vi "Read_raw_inst_setup.vi"(0 "Setup file":string) -> (8 "Setup string":string, 10 "Ch & spans choices":T2[](array[typedef]) {"Fs" format="%#_pHz"; "syncDelay" format="%#_gms"; "Ch" min=0 step=1}, 13 "PWA Data":T1, 14 "Number of Analogue instruments":i32=1, 15 "Setup filename out":string, 16 "LDA data":enum16{"No LDA data", "Take LDA data"}(ring)=enum."Take LDA data", 19 "Use Analogue channel to software sync with LDA":bool)   [LabVIEW 2022 SP3]
uses:
  Controls/Meas input Cluster.ctl
  Controls/Inst_type.ctl
  Controls/portOrDev.ctl
  Controls/calType.ctl
  Controls/channelState.ctl
  Controls/PWA_Data.ctl
  Controls/Post_Process.ctl
  File/Setup_Filetype.ctl
  Controls/Trigger_Mode.ctl
  Controls/Initial Positions.ctl
  Controls/Tunnel_Coordinates.ctl
  Globals/Meas_global.vi
  Globals/Trav_pos_global.vi
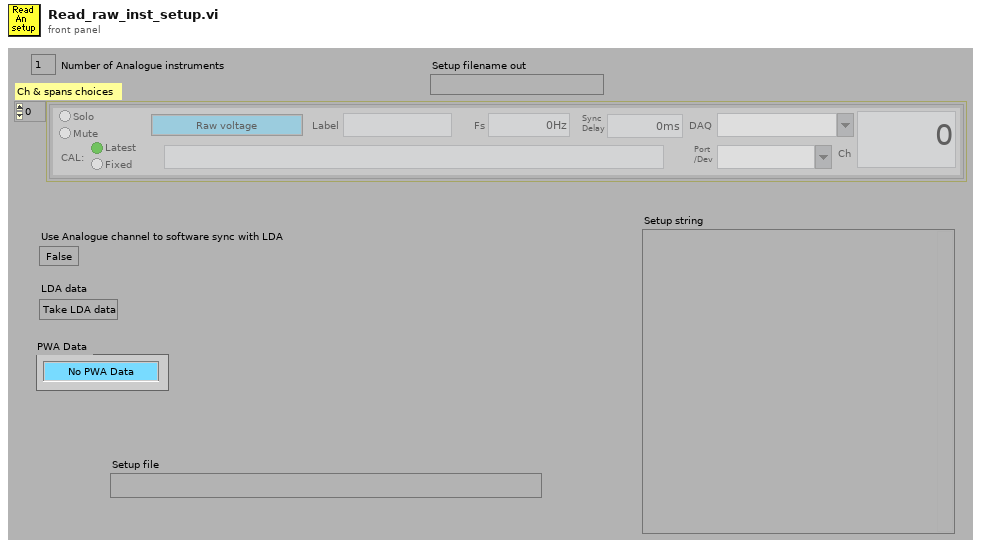
[diagram p1: front panel]
types:
  T1 = typedef "PWA_Data.ctl" = enum16{"No PWA Data", "One Ch PWA"}
  T2 = typedef "Meas input Cluster.ctl" = cluster{"Type":T3, "Label":string, "DAQ":string, "Port":T4, "Ch":i32, "Cal":path, "calType":T5, "Fs":dbl, "syncDelay":dbl, "chState":T6}
  T3 = typedef "Inst_type.ctl" = enum16{"Raw voltage", "Raw with zero offsetting", "Propeller anemometer", "Pressure Transducer", "Pitot-static tube", "Hot wire", "Cross wire 1", "Cross wire 2", "Generic Linear", "Generic Polynomial", "Generic BackPoly", "Fast FID", "Thermocouple", "Cold wire", "Pulsed Wire", "LDA Vel", "LDA Tran time", "LDA Arr time", "Microphone"}
  T4 = typedef "portOrDev.ctl" = string
  T5 = typedef "calType.ctl" = enum32{"Latest", "Fixed"}
  T6 = typedef "channelState.ctl" = enum32{"No Selection", "Solo", "Mute"}
  T7 = typedef "Post_Process.ctl" = enum16{"Take New Data", "Post Process Raw Data File"}
  T8 = typedef "Setup_Filetype.ctl" = enum16{"Measurement Setups", "Calibration Setups", "General", "Results File Plotter Setups", "Speed Calib Tweaks"}
  T9 = typedef "Trigger_Mode.ctl" = enum16{"Free Running", "Start on Trigger", "Trigger Every Block", "Trigger Every Sample"}
  T10 = typedef "Initial Positions.ctl" = cluster{"Initial XYZ":sgl[], "Traverse Setup":string, "On Axes":string, "Identity String":string}
  T11 = typedef "Tunnel_Coordinates.ctl" = enum16{"Work in Tunnel Coordinates", "Work in Model Coordinates"}
  T12 = typedef "Initial Info Cluster.ctl" = cluster{"Metadata Ch Names":string[], "Metadata Ch Values":string[]}
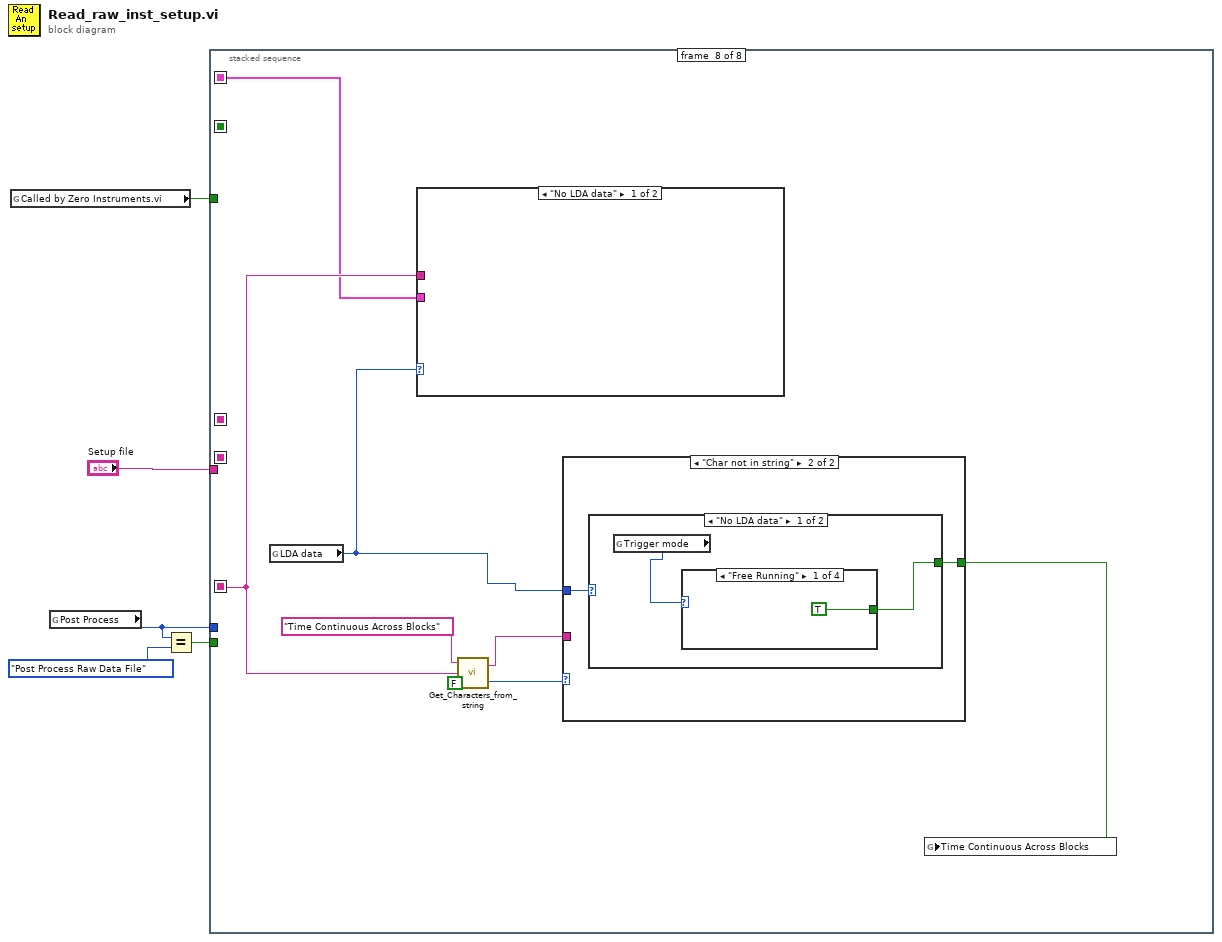
[diagram p0: block diagram]
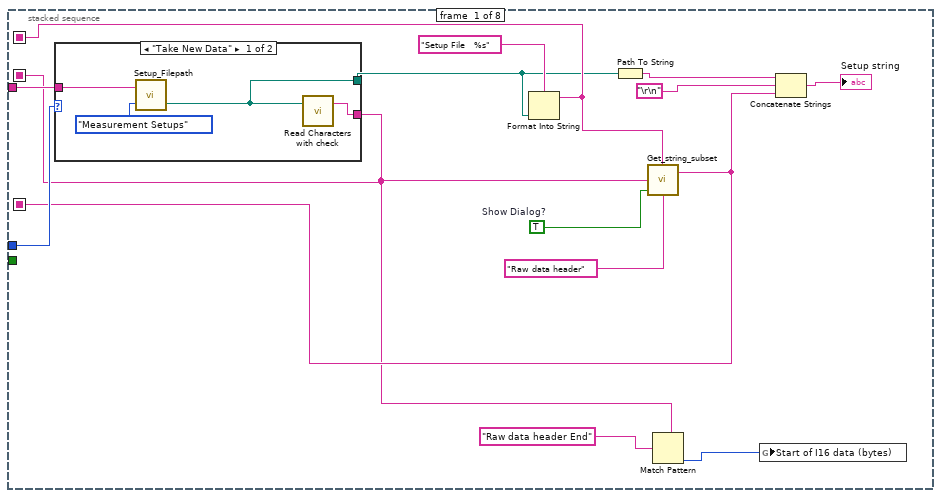
[diagram p2: hidden frame]
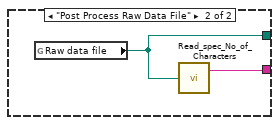
[diagram p3: hidden frame]
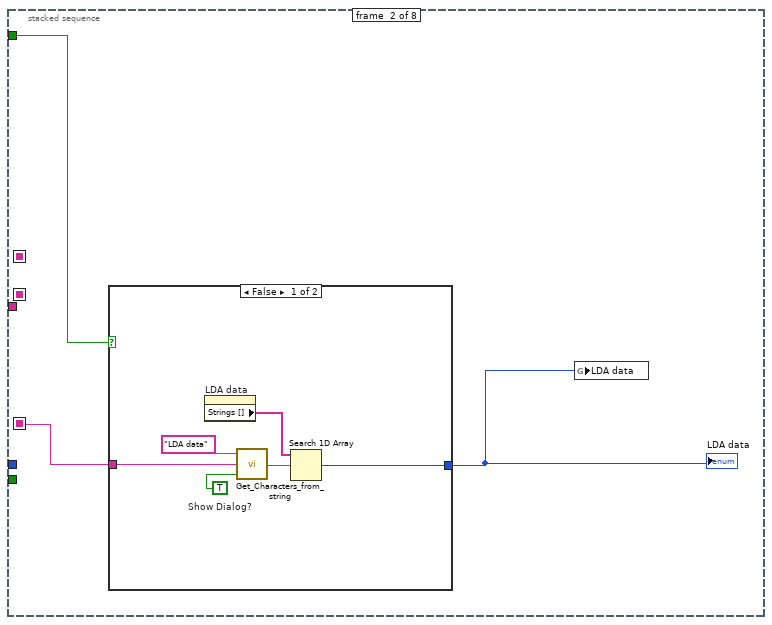
[diagram p4: hidden frame]
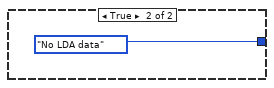
[diagram p5: hidden frame]
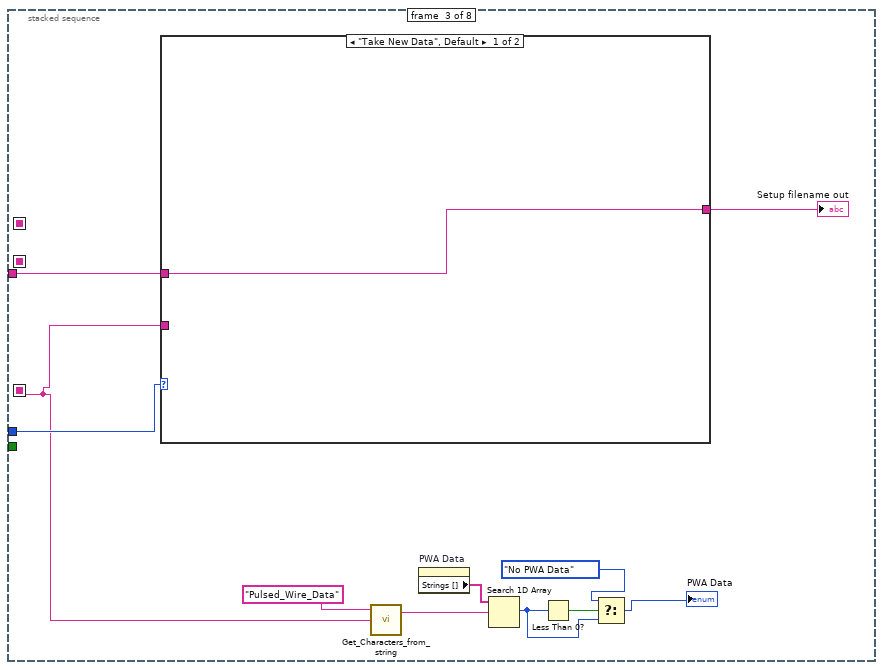
[diagram p6: hidden frame]
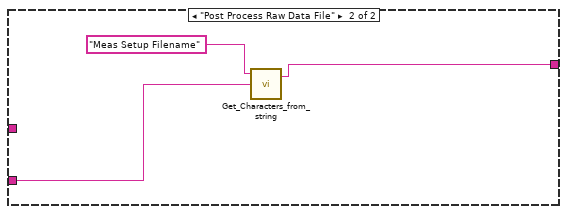
[diagram p7: hidden frame]
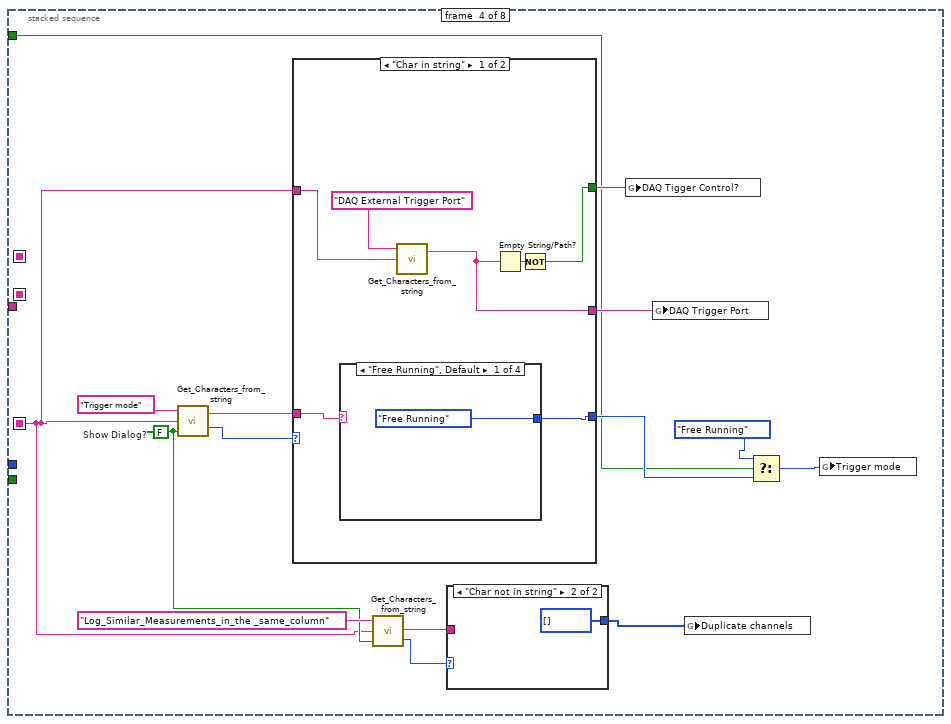
[diagram p8: hidden frame]
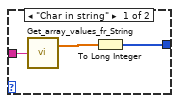
[diagram p9: hidden frame]
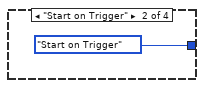
[diagram p10: hidden frame]
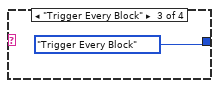
[diagram p11: hidden frame]
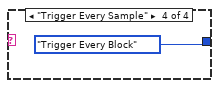
[diagram p12: hidden frame]
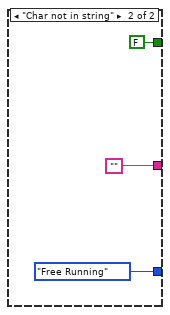
[diagram p13: hidden frame]
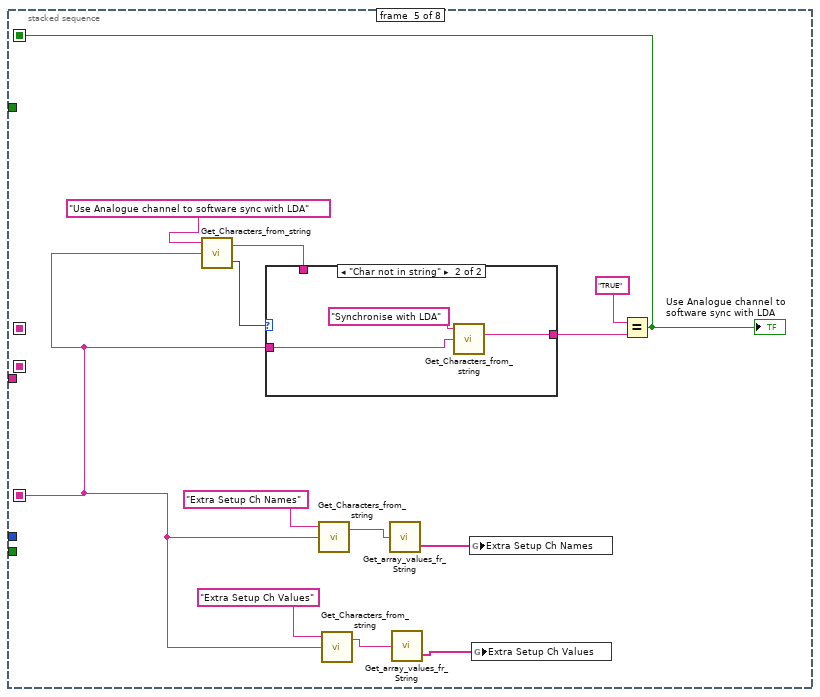
[diagram p14: hidden frame]
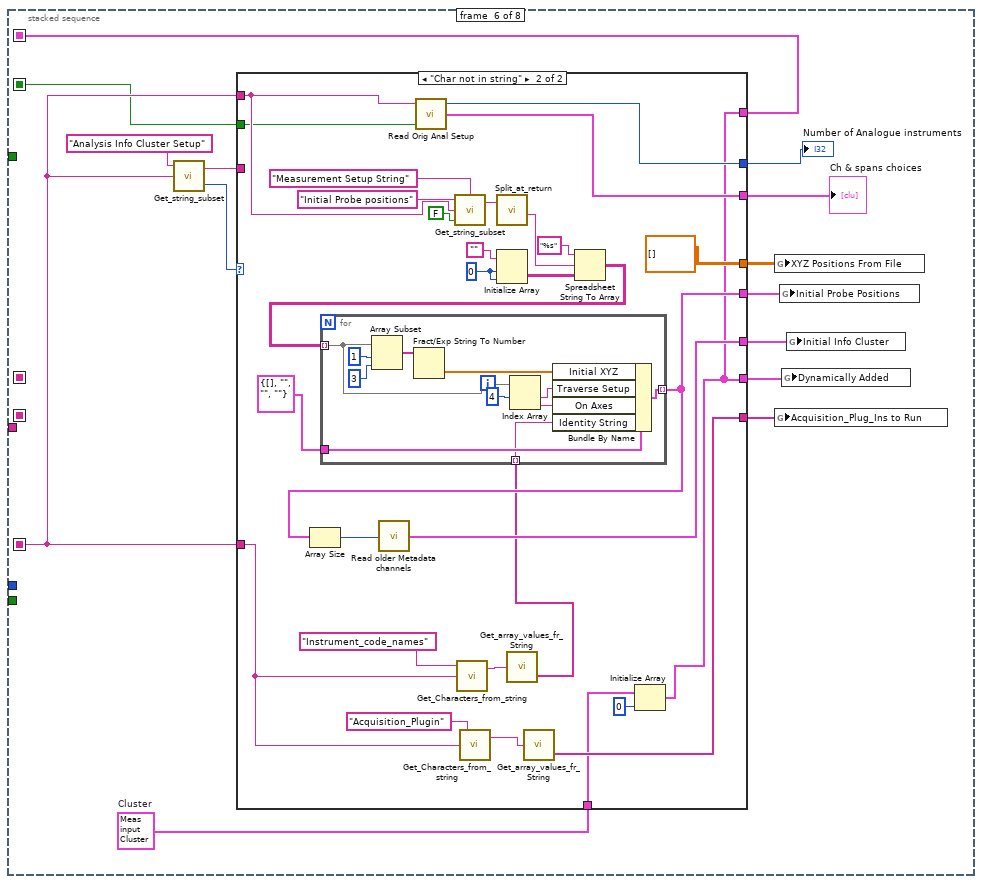
[diagram p16: hidden frame]
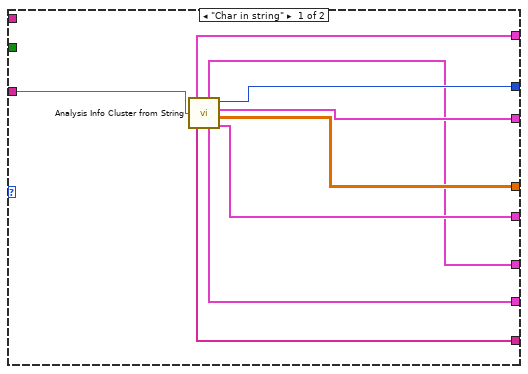
[diagram p17: hidden frame]
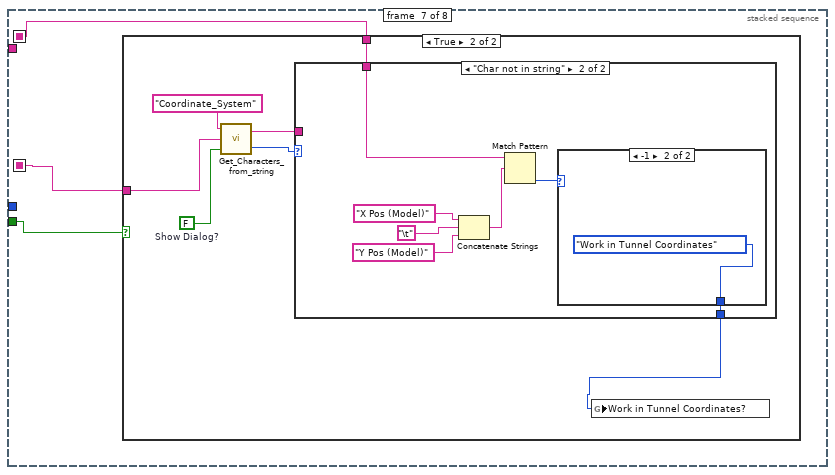
[diagram p18: hidden frame]
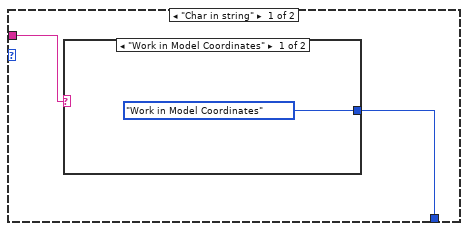
[diagram p20: hidden frame]
diagram:
  n1 = global read "Meas_global.vi" "Called by Zero Instruments.vi"() -> (w2:bool)
  n2 = global read "Meas_global.vi" "Post Process"() -> (w3:T7)
  n3 = Equal?(x=w3, y=Post_Process."Post Process Raw Data File" ("Post Process")) -> (x = y?=w5:bool)
  n4 = stacked-sequence {
    seq-local: [w8 _ _ _ _ _ _ _] -> [_ w28 w36 w57 w89 w106 w165 w188]
    seq-local: [w6 _ _ _ _ _ _ _] -> [_ _ _ _ _ _ w164 _]
    seq-local: [w11 _ _ _ _ _ _ _] -> [_ _ _ _ _ _ _ _]
    seq-local: [_ _ _ _ _ w104 _ _] -> [_ _ _ _ _ _ _ w187]
    seq-local: [_ _ _ _ w84 _ _ _] -> [_ _ _ _ _ w103 _ _]
    tunnel: w5 -> [_ _ _ _ _ _ w166 _]
    tunnel: w3 -> [w10 _ w39 _ _ _ _ _]
    tunnel: w2 -> [_ w27 _ w51 _ _ _ _]
    tunnel: "Setup file" -> [w7 _ w37 _ _ _ _ _]
    frame #0 {
      w15 = TRUE  # Show Dialog?
      n5 = case shown="\"Take New Data\"" w10 {
        tunnel: [w21 w25] -> w9
        tunnel: w7 -> [w22 _]
        tunnel: [w20 w24] -> w6
        frame "Take New Data" {
          n6 = call "Setup_Filepath.vi"("Setup File Type"=Setup_Filetype."Measurement Setups", "Filename in"=w22) -> ("Filename Out"=w21:path)  [unwired: 1 out]
          n7 = call "Read Characters with check.vi"("file (use dialog)"=w21) -> ("Read String"=w20:string)  [unwired: 1 in, 1 out]
        }
        frame "Post Process Raw Data File" {
          n8 = global read "Meas_global.vi" "Raw data file"() -> (w25:path)
          n9 = call "Read_spec_No_of_Characters.vi"("Filename"=w25) -> ("character string"=w24:string)  [unwired: 1 out]
        }
      }
      n10 = Format Into String(format string="Setup File   %s", w9) -> (resulting string=w11:string)  [unwired: 2 in, 1 out]
      n11 = Path To String(path=w9) -> (string=w16:string)
      n12 = call "Get_string_subset.vi"("String Name"=w11, "Show Dialog?"=w15, "String to split"=w6, "File Label"="Raw data header") -> ("Output string"=w8:string)  [unwired: 1 out]
      n13 = Match Pattern(string=w6, regular expression="Raw data header End") -> (offset past match=w13:i32)  [unwired: 4 out]
      n14 = global write "Meas_global.vi" "Start of I16 data (bytes)"(w13) -> ()
      n15 = Concatenate Strings(w16, "\r\n", w8) -> (→"Setup string":string)
    }
    frame #1 {
      n16 = case shown="False" w27 {
        tunnel: w28 -> [w33 _]
        tunnel: [w29 enum16{"No LDA data", "Take LDA data"}."No LDA data" ("LDA data")] -> w26
        frame False {
          w31 = TRUE  # Show Dialog?
          n17 = property on="LDA data" class="Enum (strict)"() -> ("Strings []"=w30:string[])  [unwired: 2 in, 2 out]
          n18 = call "Get_Characters_from_string.vi"("Show Dialog?"=w31, "Input string"=w33, "Variable name"="LDA data" ("Label for characters")) -> ("Value"=w34:string)  [unwired: 1 out]
          n19 = Search 1D Array(1D array=w30, element=w34) -> (index of element=w29:i32)  [unwired: 1 out]
        }
        frame True {
        }
      }
      "LDA data" <- w26
      n20 = global write "Meas_global.vi" "LDA data"(w26) -> ()
    }
    frame #2 {
      n21 = case shown="\"Take New Data\", Default" w39 {
        tunnel: [w47 w48] -> w38
        tunnel: w37 -> [w47 _]
        tunnel: w36 -> [_ w50]
        frame "Take New Data", Default {
        }
        frame "Post Process Raw Data File" {
          n22 = call "Get_Characters_from_string.vi"("Input string"=w50, "Variable name"="Meas Setup Filename" ("Label for characters")) -> ("Value"=w48:string)  [unwired: 1 in, 1 out]
        }
      }
      "Setup filename out" <- w38
      n23 = call "Get_Characters_from_string.vi"("Input string"=w36, "Variable name"="Pulsed_Wire_Data") -> ("Value"=w44:string)  [unwired: 1 in, 1 out]
      n24 = property on="PWA Data" class="Enum (strict)"() -> ("Strings []"=w45:string[])  [unwired: 2 in, 2 out]
      n25 = Search 1D Array(1D array=w45, element=w44) -> (index of element=w41:i32)  [unwired: 1 out]
      n26 = Less Than 0?(x=w41) -> (x < 0?=w43:bool)
      n27 = Select(t=PWA_Data."No PWA Data" ("PWA Data"), s=w43, f=w41) -> (s? t:f=→"PWA Data":i32)
    }
    frame #3 {
      w61 = FALSE  # Show Dialog?
      n28 = call "Get_Characters_from_string.vi"("Show Dialog?"=w61, "Input string"=w57, "Variable name"="Trigger mode") -> ("Status"=w64:enum16{"Char in string", "Char not in string"}, "Value"=w63:string)
      n29 = case shown="\"Char in string\"" w64 {
        tunnel: [w75 Trigger_Mode."Free Running" ("Trigger mode")] -> w54
        tunnel: w63 -> [w76 _]
        tunnel: w57 -> [w73 _]
        tunnel: [w70 FALSE] -> w56
        tunnel: [w72 ""] -> w55
        frame "Char in string" {
          n30 = case shown="\"Free Running\", Default" w76 {
            tunnel: [Trigger_Mode."Free Running" ("Trigger mode") Trigger_Mode."Start on Trigger" ("Trigger mode") Trigger_Mode."Trigger Every Block" ("Trigger mode") Trigger_Mode."Trigger Every Block" ("Trigger mode")] -> w75
            frame "Free Running", Default {
            }
            frame "Start on Trigger" {
            }
            frame "Trigger Every Block" {
            }
            frame "Trigger Every Sample" {
            }
          }
          n31 = call "Get_Characters_from_string.vi"("Input string"=w73, "Variable name"="DAQ External Trigger Port") -> ("Value"=w72:string)  [unwired: 1 in, 1 out]
          n32 = Empty String/Path?(string/path=w72) -> (empty?=w71:bool)
          n33 = Not(x=w71) -> (.not. x?=w70:bool)
        }
        frame "Char not in string" {
        }
      }
      n34 = call "Get_Characters_from_string.vi"("Show Dialog?"=w61, "Input string"=w57, "Variable name"="Log_Similar_Measurements_in_the _same_column") -> ("Status"=w58:enum16{"Char in string", "Char not in string"}, "Value"=w60:string)
      n35 = case shown="\"Char not in string\"" w58 {
        tunnel: w60 -> [w68 _]
        tunnel: [w66 i32[] []] -> w59
        frame "Char in string" {
          n36 = call "Get_array_values_fr_String.vi"("String Value"=w68) -> ("Numeric Array"=w67:dbl[])  [unwired: 1 out]
          n37 = To Long Integer(number=w67) -> (32bit integer=w66:i32[])
        }
        frame "Char not in string" {
        }
      }
      n38 = global write "Meas_global.vi" "DAQ Tigger Control?"(w56) -> ()
      n39 = global write "Meas_global.vi" "DAQ Trigger Port"(w55) -> ()
      n40 = global write "Meas_global.vi" "Duplicate channels"(w59) -> ()
      n41 = Select(t=Trigger_Mode."Free Running" ("Trigger mode"), s=w51, f=w54) -> (s? t:f=w53:T9)
      n42 = global write "Meas_global.vi" "Trigger mode"(w53) -> ()
    }
    frame #4 {
      n43 = call "Get_Characters_from_string.vi"("Input string"=w89, "Variable name"="Use Analogue channel to software sync with LDA") -> ("Status"=w95:enum16{"Char in string", "Char not in string"}, "Value"=w94:string)  [unwired: 1 in]
      n44 = case shown="\"Char not in string\"" w95 {
        tunnel: w89 -> [_ w100]
        tunnel: [w97 w98] -> w96
        tunnel: w94 -> [w97 _]
        frame "Char in string" {
        }
        frame "Char not in string" {
          n45 = call "Get_Characters_from_string.vi"("Input string"=w100, "Variable name"="Synchronise with LDA") -> ("Value"=w98:string)  [unwired: 1 in, 1 out]
        }
      }
      n46 = call "Get_Characters_from_string.vi"("Input string"=w89, "Variable name"="Extra Setup Ch Names") -> ("Value"=w88:string)  [unwired: 1 in, 1 out]
      n47 = call "Get_Characters_from_string.vi"("Input string"=w89, "Variable name"="Extra Setup Ch Values") -> ("Value"=w87:string)  [unwired: 1 in, 1 out]
      n48 = call "Get_array_values_fr_String.vi"("String Value"=w88) -> ("String array"=w85:string[])  [unwired: 1 out]
      n49 = call "Get_array_values_fr_String.vi"("String Value"=w87) -> ("String array"=w86:string[])  [unwired: 1 out]
      n50 = global write "Meas_global.vi" "Extra Setup Ch Names"(w85) -> ()
      n51 = global write "Meas_global.vi" "Extra Setup Ch Values"(w86) -> ()
      n52 = Equal?(x="TRUE", y=w96) -> (x = y?=w84:bool)
      "Use Analogue channel to software sync with LDA" <- w84
    }
    frame #5 {
      w101 = T2 {"Type"=enum."Raw voltage", "Label"="", "DAQ"="", "Port"="", "Ch"=0, "Cal"=path "", "calType"=enum."Latest", "Fs"=0.0, "syncDelay"=0.0, "chState"=enum."No Selection"}  # Cluster
      n53 = call "Get_string_subset.vi"("String to split"=w106, "File Label"="Analysis Info Cluster Setup") -> ("Status"=w113:enum16{"Char in string", "Char not in string"}, "Output string"=w110:string)  [unwired: 2 in]
      n54 = case shown="\"Char not in string\"" w113 {
        tunnel: w106 -> [_ w140]
        tunnel: [w122 w152] -> w112
        tunnel: [w121 w151] -> w111
        tunnel: w110 -> [w123 _]
        tunnel: [w120 w137] -> w109
        tunnel: [w119 dbl[][] [] ("XYZ Positions")] -> w108
        tunnel: [w118 w135] -> w107
        tunnel: w106 -> [_ w129]
        tunnel: [w117 w128] -> w105
        tunnel: [w116 w124] -> w104
        tunnel: w103 -> [_ w127]
        tunnel: [w115 w124] -> w102
        tunnel: w101 -> [_ w126]
        frame "Char in string" {
          n55 = call "Analysis Info Cluster from String.vi"("Setup String"=w123) -> ("Initial Probe Positions"=w120:T10[], "Dynamically Added"=w115:T2[], "XYZ Positions"=w119:dbl[][], "Ch & spans choices"=w122:T2[], "Initial Info Cluster"=w118:T12[], "Number of Analogue instruments"=w121:i32, "Acquisition_Plugin"=w117:string[], "LDA Setup"=w116:T2[])
        }
        frame "Char not in string" {
          w143 = 0 ("Dimension Size")
          n56 = call "Read Orig Anal Setup.vi"("Use Analogue channel to software sync with LDA"=w127, "Setup string"=w140) -> ("Ch & spans choices"=w152:T2[], "Number of Analogue instruments"=w151:i32)  [unwired: 2 in]
          n57 = call "Get_string_subset.vi"("String Name"="Measurement Setup String", "Show Dialog?"=FALSE, "String to split"=w140, "File Label"="Initial Probe positions") -> ("Output string"=w141:string)  [unwired: 1 out]
          n58 = call "Get_Characters_from_string.vi"("Input string"=w129, "Variable name"="Instrument_code_names") -> ("Value"=w134:string)  [unwired: 1 in, 1 out]
          n59 = call "Get_Characters_from_string.vi"("Input string"=w129, "Variable name"="Acquisition_Plugin") -> ("Value"=w131:string)  [unwired: 1 in, 1 out]
          n60 = call "Split_at_return.vi"("String"=w141) -> ("after substring"=w146:string)  [unwired: 1 in, 3 out]
          n61 = Initialize Array("", w143, w143) -> (w142:string[][])
          n62 = call "Get_array_values_fr_String.vi"("String Value"=w134) -> ("String array"=w132:string[])  [unwired: 1 out]
          n63 = call "Get_array_values_fr_String.vi"("String Value"=w131) -> ("String array"=w128:string[])  [unwired: 1 out]
          n64 = Spreadsheet String To Array(format string="%s", spreadsheet string=w146, array type (2D Dbl)=w142) -> (array=w139:string[][])  [unwired: 1 out]
          n65 = for {
            tunnel: w139 -> [w158] mode=indexing
            tunnel: T10 {"Initial XYZ"=[], "Traverse Setup"="", "On Axes"="", "Identity String"=""} ("Initial Positions 3") -> [w161]
            tunnel: [w154] -> w137 mode=indexing
            tunnel: w132 -> [w153] mode=indexing
            n66 = Array Subset(array=w158, index=1, length=3) -> (w160:string[])
            n67 = Fract/Exp String To Number(string=w160) -> (number=w159:dbl[])  [unwired: 3 in, 1 out]
            n68 = Index Array(array=w158, index #1=4 ("index")) -> (element #1=w156:string, element #2=w155:string)  [unwired: 1 in]
            n69 = Bundle By Name(cluster=w161, "Initial XYZ"=w159, "Traverse Setup"=w156, "On Axes"=w155, "Identity String"=w153) -> (w154:T10)
          }
          n70 = Array Size(array=w137) -> (size(s)=w136:i32)
          n71 = call "Read older Metadata channels.vi"("Number of Channels"=w136) -> ("Initial Info Cluster"=w135:T12[])
          n72 = Initialize Array(w126, 0 ("dimension size")) -> (w124:T2[])
        }
      }
      "Ch & spans choices" <- w112
      "Number of Analogue instruments" <- w111
      n73 = global write "Meas_global.vi" "XYZ Positions From File"(w108) -> ()
      n74 = global write "Meas_global.vi" "Acquisition_Plug_Ins to Run"(w105) -> ()
      n75 = global write "Meas_global.vi" "Initial Probe Positions"(w109) -> ()
      n76 = global write "Meas_global.vi" "Dynamically Added"(w102) -> ()
      n77 = global write "Meas_global.vi" "Initial Info Cluster"(w107) -> ()
    }
    frame #6 {
      n78 = case shown="True" w166 {
        tunnel: w165 -> [_ w172]
        tunnel: w164 -> [_ w167]
        frame False {
        }
        frame True {
          w171 = FALSE  # Show Dialog?
          n79 = call "Get_Characters_from_string.vi"("Show Dialog?"=w171, "Input string"=w172, "Variable name"="Coordinate_System" ("Label for characters")) -> ("Status"=w170:enum16{"Char in string", "Char not in string"}, "Value"=w169:string)
          n80 = case shown="\"Char not in string\"" w170 {
            tunnel: w169 -> [w175 _]
            tunnel: [w174 w178] -> w168
            tunnel: w167 -> [_ w180]
            frame "Char in string" {
              n81 = case shown="\"Work in Model Coordinates\"" w175 {
                tunnel: [Tunnel_Coordinates."Work in Model Coordinates" ("Work in Tunnel Coordinates?") Tunnel_Coordinates."Work in Tunnel Coordinates" ("Work in Tunnel Coordinates?")] -> w174
                frame "Work in Model Coordinates" {
                }
                frame "Work in Tunnel Coordinates", Default {
                }
              }
            }
            frame "Char not in string" {
              n82 = Concatenate Strings("X Pos (Model)", "\t", "Y Pos (Model)") -> (w181:string)
              n83 = Match Pattern(string=w180, regular expression=w181) -> (offset past match=w179:i32)  [unwired: 4 out]
              n84 = case shown="-1" w179 {
                tunnel: [Tunnel_Coordinates."Work in Model Coordinates" ("Work in Tunnel Coordinates?") Tunnel_Coordinates."Work in Tunnel Coordinates" ("Work in Tunnel Coordinates?")] -> w178
                frame 0, Default {
                }
                frame -1 {
                }
              }
            }
          }
          n85 = global write "Trav_pos_global.vi" "Work in Tunnel Coordinates?"(w168) -> ()
        }
      }
    }
    frame #7 {
      n86 = global read "Meas_global.vi" "LDA data"() -> (w189:enum16{"No LDA data", "Take LDA data"})
      n87 = case shown="\"No LDA data\"" w189 {
        tunnel: w188 -> [_ w196]
        tunnel: w187 -> [_ w195]
        frame "No LDA data" {
        }
        frame "Take LDA data" {
          n88 = call "Load_LDA_Channel_Setup.vi"("LDA Setup"=w195, "Setup file string"=w196) -> ()  [unwired: 1 in]
        }
      }
      n89 = call "Get_Characters_from_string.vi"("Show Dialog?"=FALSE, "Input string"=w188, "Variable name"="Time Continuous Across Blocks") -> ("Status"=w192:enum16{"Char in string", "Char not in string"}, "Value"=w190:string)
      n90 = case shown="\"Char not in string\"" w192 {
        tunnel: [w197 w201] -> w191
        tunnel: w190 -> [w199 _]
        tunnel: w189 -> [_ w200]
        frame "Char in string" {
          n91 = Equal?(x="TRUE", y=w199) -> (x = y?=w197:bool)
        }
        frame "Char not in string" {
          n92 = case shown="\"No LDA data\"" w200 {
            tunnel: [w202 FALSE ("Time Continuous Across Blocks")] -> w201
            frame "No LDA data" {
              n93 = global read "Meas_global.vi" "Trigger mode"() -> (w203:T9)
              n94 = case shown="\"Free Running\"" w203 {
                tunnel: [TRUE TRUE FALSE FALSE] -> w202
                frame "Free Running" {
                }
                frame "Start on Trigger" {
                }
                frame "Trigger Every Block" {
                }
                frame "Trigger Every Sample" {
                }
              }
            }
            frame "Take LDA data" {
            }
          }
        }
      }
      n95 = global write "Meas_global.vi" "Time Continuous Across Blocks"(w191) -> ()
    }
  }
